vi "Dust UI.vi"() -> ()   [LabVIEW 2009, in "UI.lvlib"]
uses:
  UI.lvlib
panel:
  in  "stop":bool
  in  "Dust Definitions":i32(listbox)
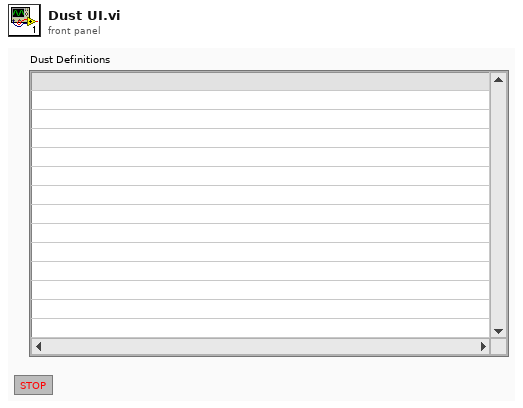
[diagram p1: front panel]
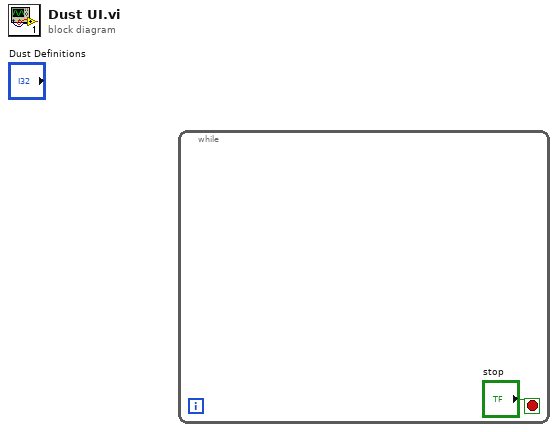
[diagram p0: block diagram]
diagram:
  n1 = while {
    stop <- "stop" stop-if-true
  }
